vi "Deposit.vi"   [LabVIEW 2013, in "ToplevelControllerLibrary.lvlib"]
uses:
  ToplevelControllerLibrary.lvlib
  Private Controls/Deposit.ctl
types:
  T1 = typedef "ToplevelControllerLibrary.lvlib/Deposit.ctl" = enum16{"Deposit", "Monitor SensorConsole", "Update DB", "Idle"}
  T2 = enum16{"Init", "Enqueue", "Dequeue", "ReleaseQueue", "Exit"}
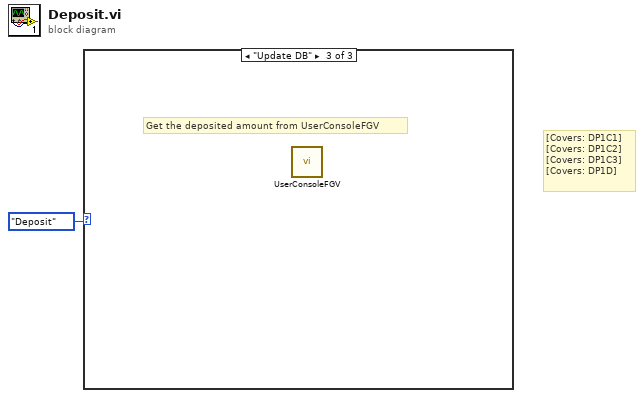
[diagram p0: block diagram]
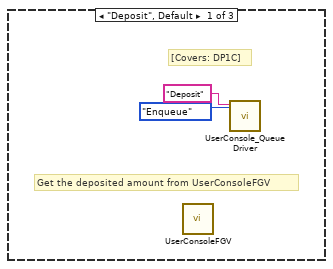
[diagram p2: hidden frame]
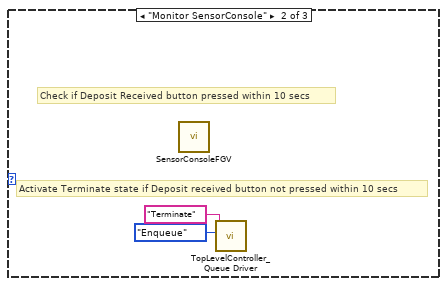
[diagram p3: hidden frame]
diagram:
  # "[Covers: DP1C1] \n[Covers: DP1C2] \n[Covers: DP1C3] \n[Covers: DP1D]"
  n1 = case shown="\"Update DB\"" Deposit."Deposit" {
    frame "Deposit", Default {
      # "Get the deposited amount from UserConsoleFGV"
      # "[Covers: DP1C]"
      n2 = call "UserConsoleFGV.vi"() -> ()  [unwired: 10 in, 2 out]
      n3 = call "UserConsole_Queue Driver.vi"("State"=T2."Enqueue" ("Enum"), "EnQ"="Deposit") -> ()  [unwired: 8 in, 2 out]
    }
    frame "Monitor SensorConsole" {
      # "Activate Terminate state if Deposit received button not pressed within 10 secs"
      # "Check if Deposit Received button pressed within 10 secs"
      n4 = call "SensorConsoleFGV.vi"() -> ()  [unwired: 10 in, 2 out]
      n5 = call "TopLevelController_Queue Driver.vi"("Enum"=T2."Enqueue", "EnQ"="Terminate") -> ()  [unwired: 8 in, 2 out]
    }
    frame "Update DB" {
      # "Get the deposited amount from UserConsoleFGV"
      n6 = call "UserConsoleFGV.vi"() -> ()  [unwired: 10 in, 2 out]
    }
  }
